vi "Wavelength set.vi"(8 "error in (no error)":errorcluster, 10 "Wavelength (nnnn)":dbl[unit], 11 "VISA resource name":refnum<visa-resource-name>) -> (0 "error out":errorcluster, 3 "VISA resource name out":refnum<visa-resource-name>)   [LabVIEW 2013, in "Newport 1830-C.lvlib"]
doc: "Four integers are digits of wavelength in nm\nlmno"
uses:
  Newport 1830-C.lvlib
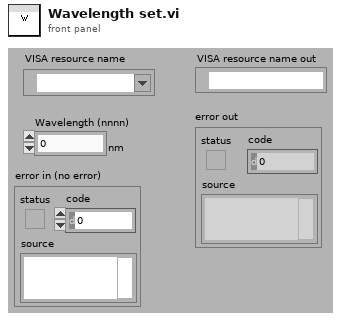
[diagram p1: front panel]
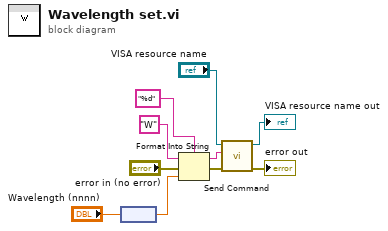
[diagram p0: block diagram]
diagram:
  n1 = node("Wavelength (nnnn)") -> (w1:dbl)
  n2 = Format Into String(format string="%d", initial string="W" ("command"), error in="error in (no error)", w1) -> (resulting string=w3:string, error out=w4:errorcluster)
  n3 = call "Send Command.vi"("error in (no error)"=w4, "write buffer"=w3, "VISA resource name In"="VISA resource name") -> ("error out"=→"error out":errorcluster, "VISA resource name out"=→"VISA resource name out":refnum<visa-resource-name>)  [unwired: 7 in]
